vi "LS DAS Loop.vi"(11 "FPGA Ref":refnum<k20>) -> ()   [LabVIEW 2019]
uses:
  <vilib>/Utility/error.llb/Error Cluster From Error Code.vi
  <vilib>/rvi/errors/niLvFpgaAdjustHostInterfaceError.vi
  <vilib>/rvi/interface/nirviMethod/nirviMethod.xnode
  FPGA Bitfiles/LS_Acquisition_FPGA_9627.lvbitx
  <vilib>/rvi/errors/niLvFpgaMergeErrorWithErrorCode.vi
  <vilib>/FPGAPlugInAG/sbRIO-9627/niLvFpga_ReadFifo_sbRIO-9627.vi
panel:
  out "FIFO loops":i32
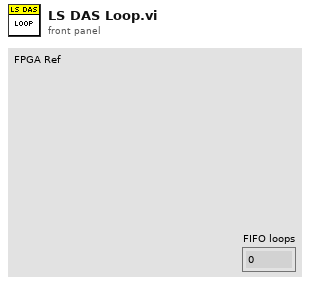
[diagram p1: front panel]
types:
  T1 = cluster{"FPGA Ref":refnum<k20>, "Time":dbl, "PtsTaken":i32, "Pts/File":i32, "10AveWait":u32, "Bank1 Filepath":path, "FileIndex":i32, "FilesUsed":i32, "Day":i32, "Bank2 Filepath":path, "DataCount":i32, "Note":string, "Anomaly Filepath":path, "File2 DataCount":i32}
  T2 = enum16{"Read", "Engine Writes", "Main Writes", "Write Anomalies", "Write Init Data", "Write Storage", "Write Note", "Read Note"}
  T3 = enum16{"open", "replace", "create", "open or create", "replace or create", "replace or create with confirmation"}
  T4 = typedef "LS Data.ctl" = cluster{"Total Cycles":u32[], "Steps":u32[], "Anomalies Total":i32[], "Cycles":u32[], "Anomalies/Cycle":i32[], "Anomalies (Last Cycle)":i32[], "Opens":i32[]}
  T5 = cluster{"Running?":bool, "Record":bool, "Data Filepath":path, "Serial Numbers":string[]}
  T6 = typedef "LVDateTimeRec.ctl" = cluster{"fractional second":dbl, "second":i32, "minute":i32, "hour":i32, "day of month":i32, "month":i32, "year":i32, "day of week":i32, "day of year":i32, "DST":i32}
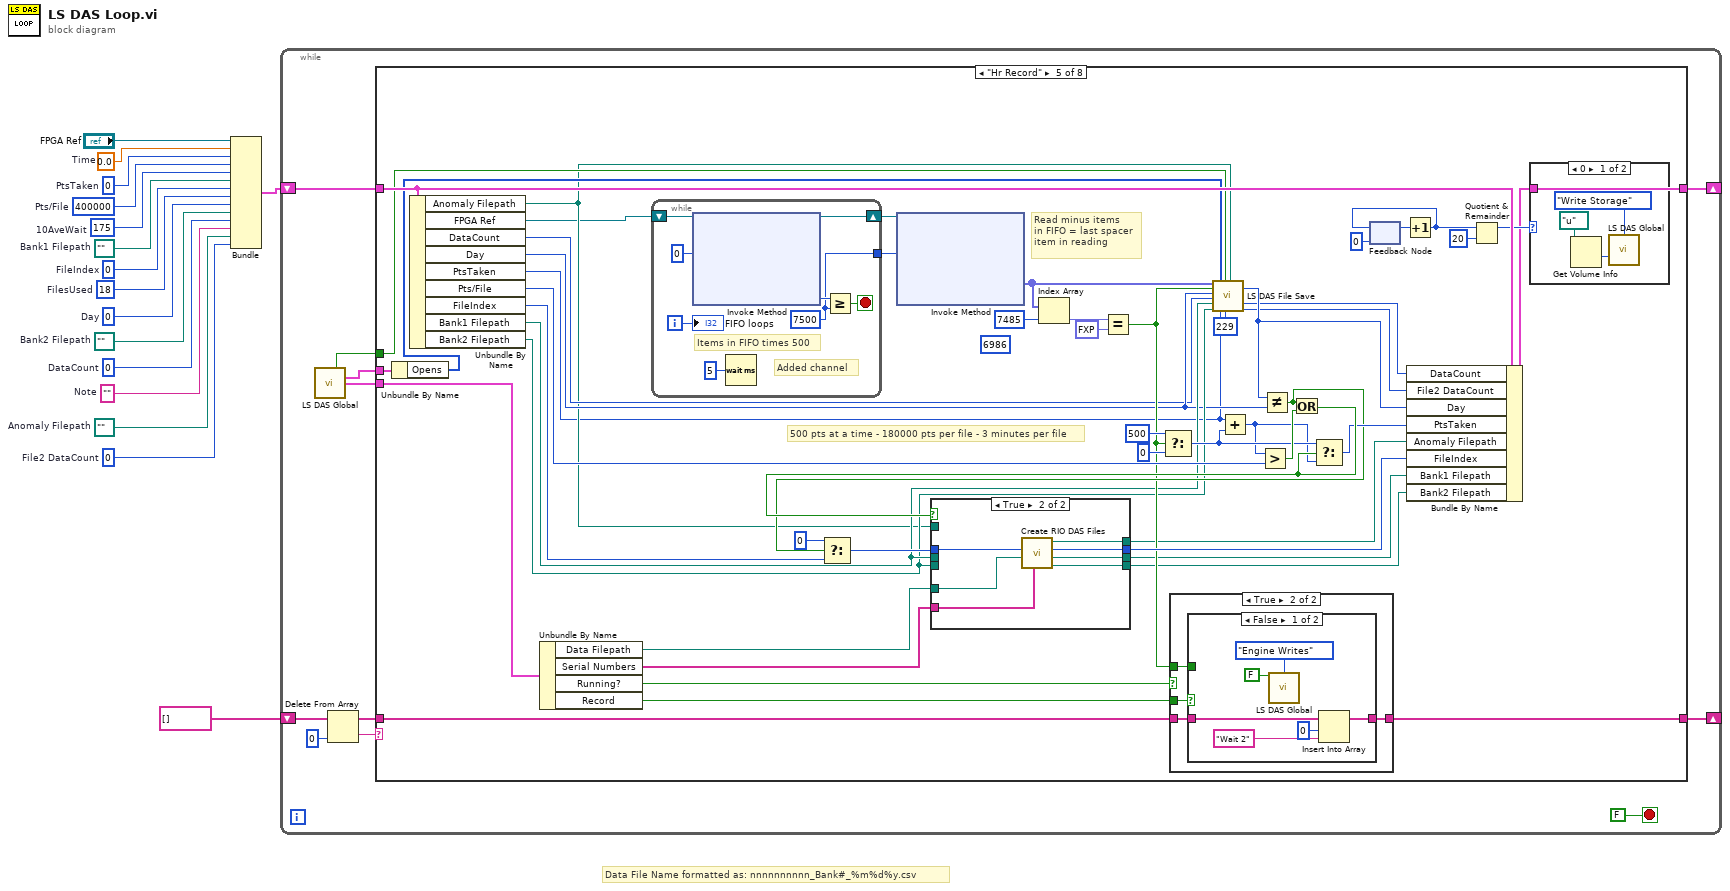
[diagram p0: block diagram]
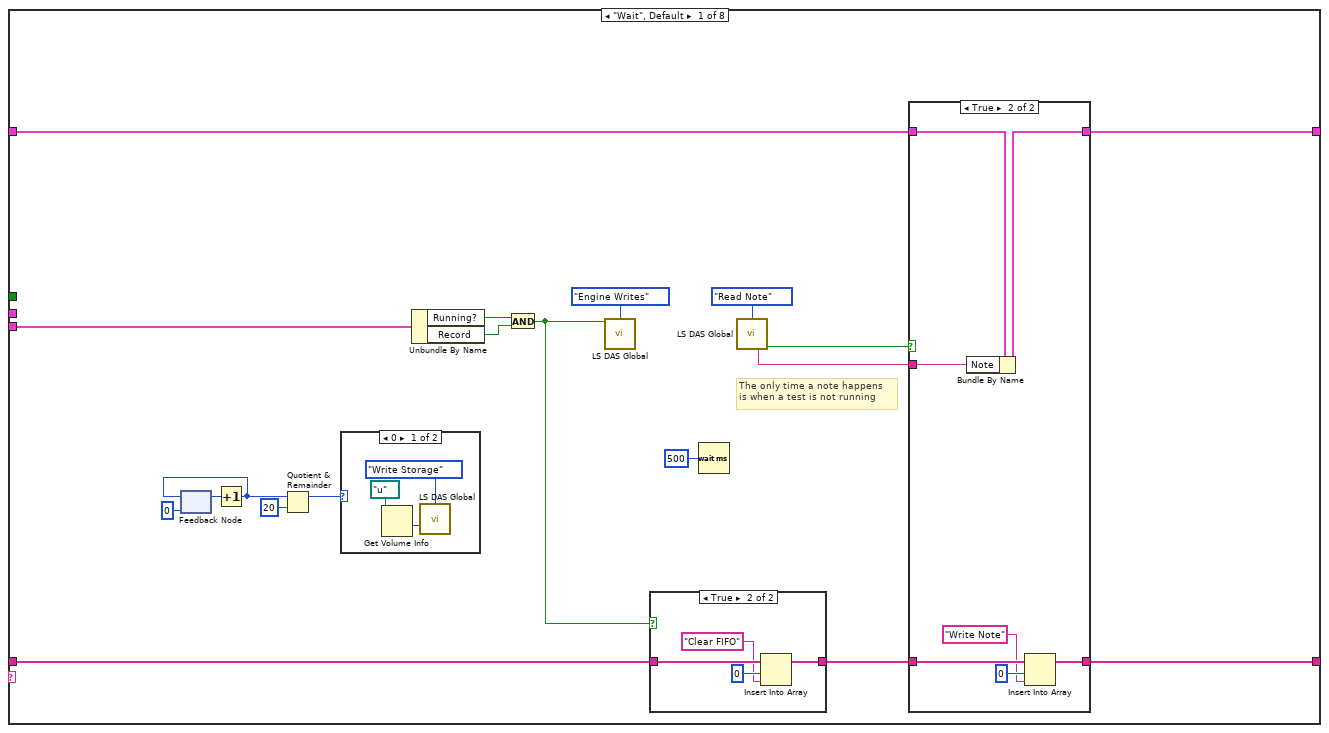
[diagram p2: hidden frame]
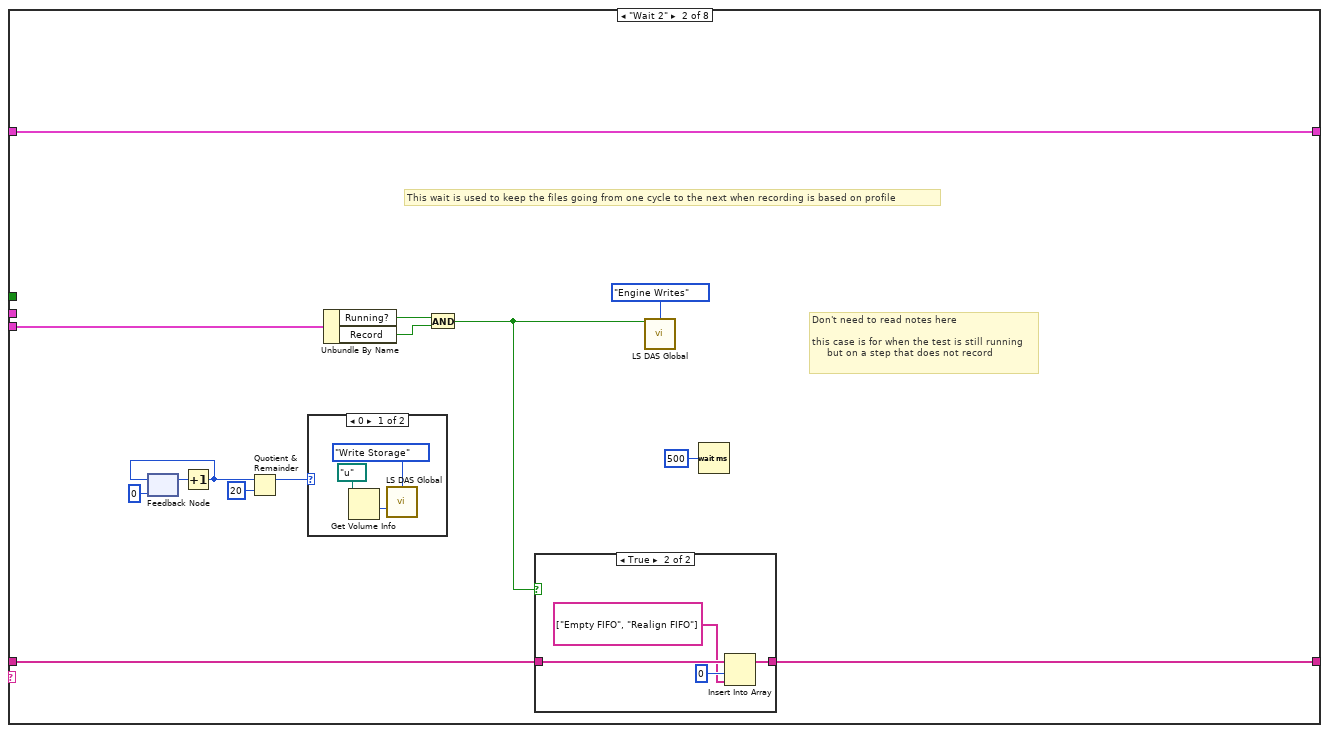
[diagram p6: hidden frame]
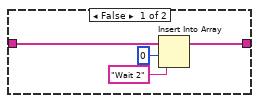
[diagram p8: hidden frame]
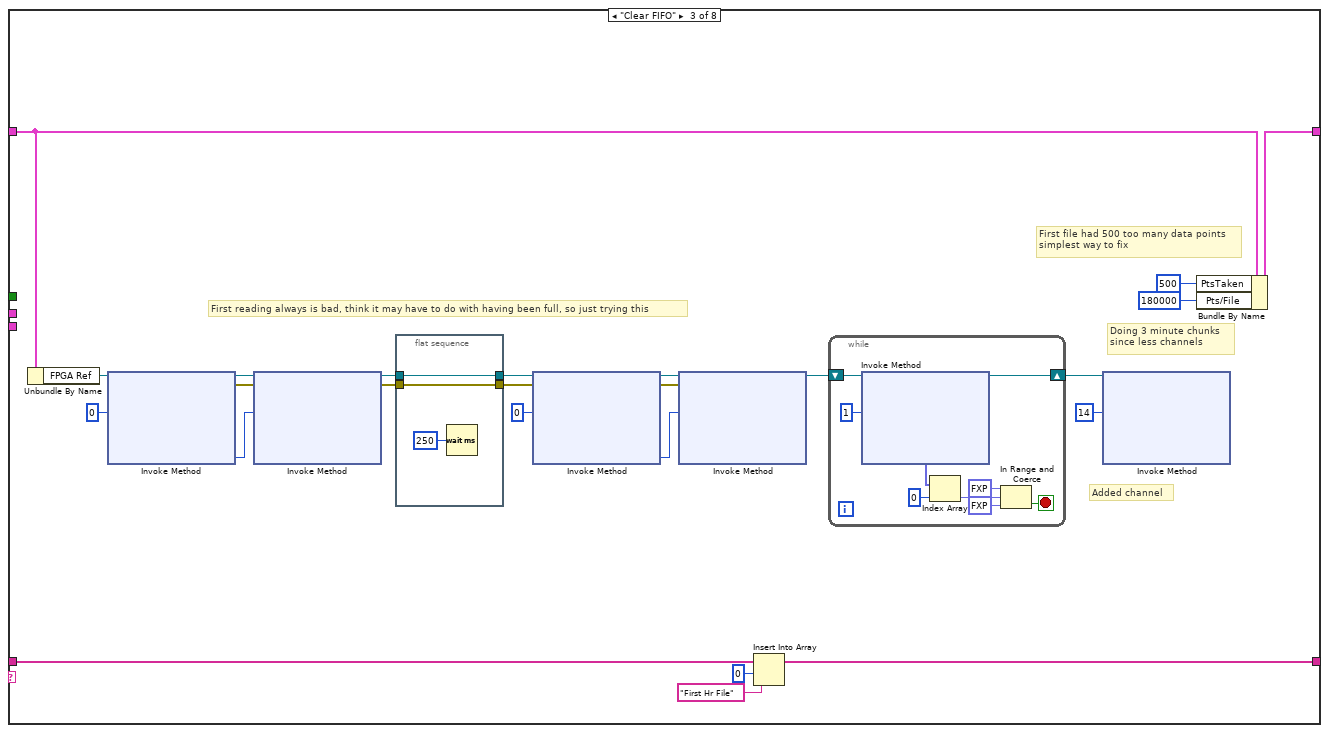
[diagram p9: hidden frame]
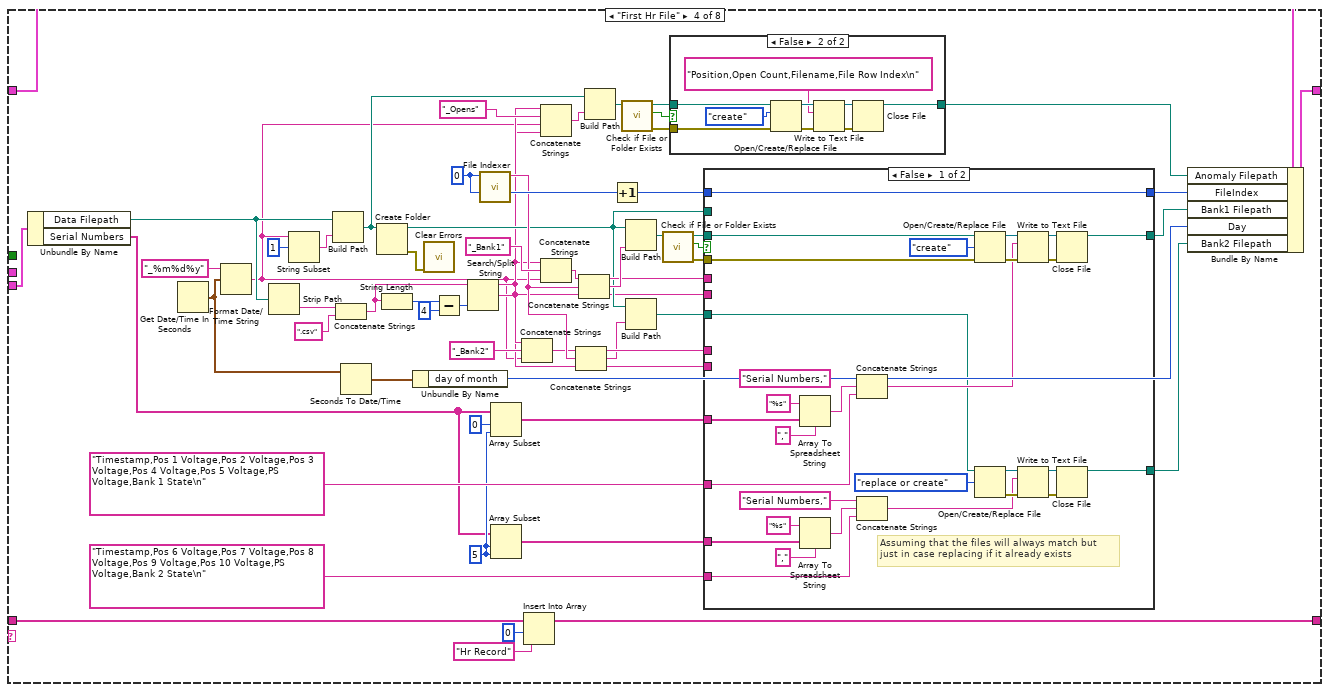
[diagram p10: hidden frame]
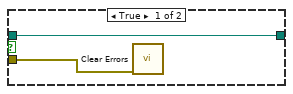
[diagram p11: hidden frame]
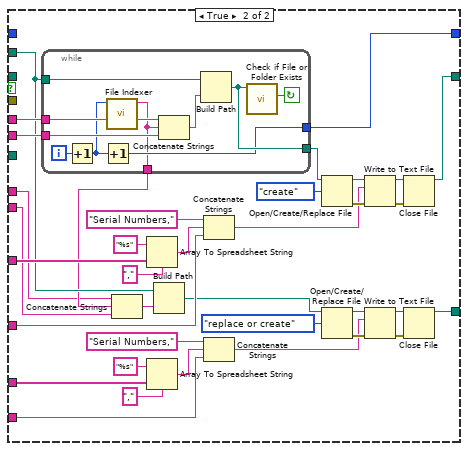
[diagram p12: hidden frame]
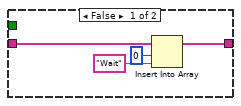
[diagram p14: hidden frame]
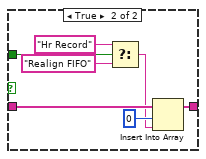
[diagram p15: hidden frame]
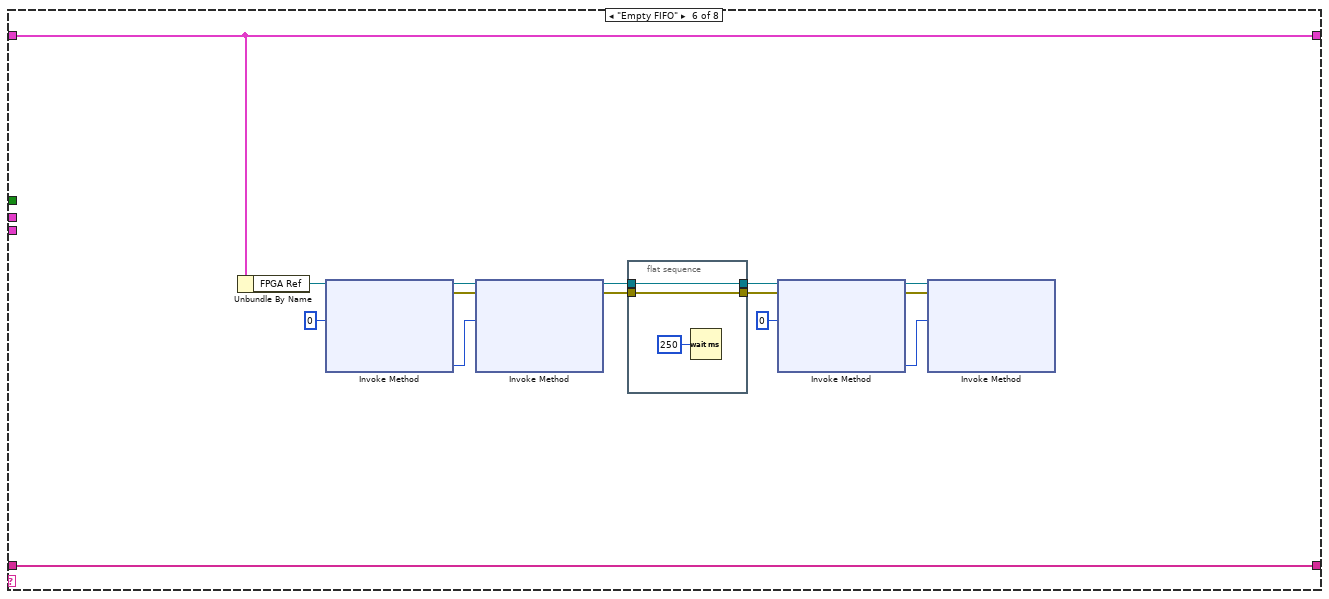
[diagram p17: hidden frame]
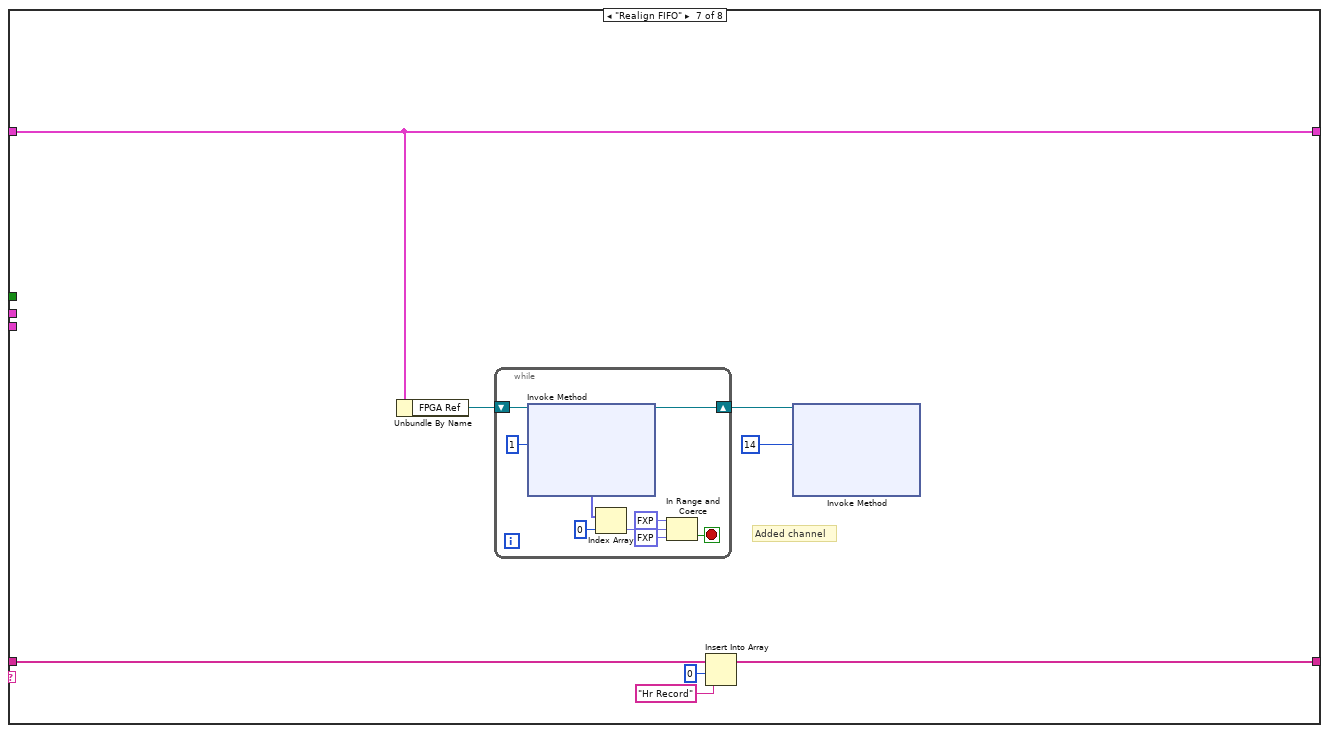
[diagram p18: hidden frame]
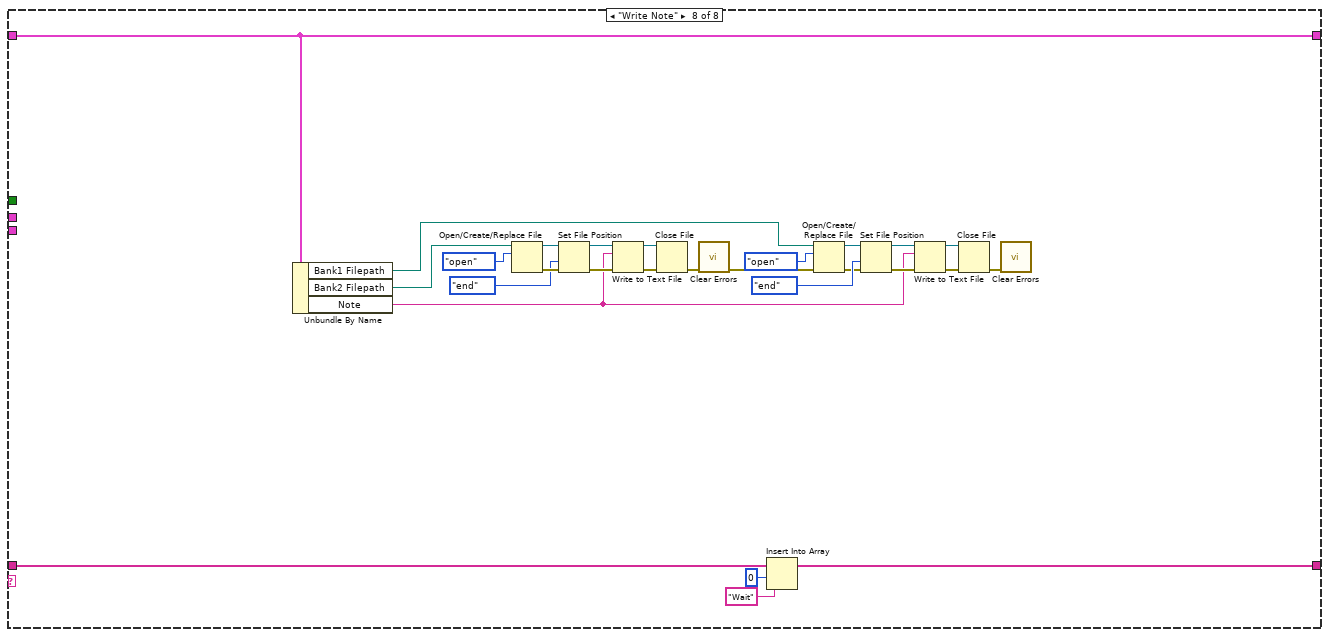
[diagram p19: hidden frame]
diagram:
  w2 = 0  # File2 DataCount
  w3 = path ""  # Anomaly Filepath
  w4 = ""  # Note
  w5 = 0  # DataCount
  w6 = path ""  # Bank2 Filepath
  w7 = 0  # Day
  w8 = 18  # FilesUsed
  w9 = 0  # FileIndex
  w10 = path ""  # Bank1 Filepath
  w11 = u32 175  # 10AveWait
  w12 = 400000  # Pts/File
  w13 = 0  # PtsTaken
  w16 = 0.0  # Time
  # "Data File Name formatted as: nnnnnnnnnn_Bank#_%m%d%y.csv"
  n1 = Bundle("FPGA Ref"="FPGA Ref", "Time"=w16, "PtsTaken"=w13, "Pts/File"=w12, "10AveWait"=w11, "Bank1 Filepath"=w10, "FileIndex"=w9, "FilesUsed"=w8, "Day"=w7, "Bank2 Filepath"=w6, "DataCount"=w5, "Note"=w4, "Anomaly Filepath"=w3, "File2 DataCount"=w2) -> (w15:T1)  [unwired: 1 in]
  n2 = while {
    shift-right: [w25] -> _
    shift-left: w15 -> [w26]
    shift-right: [w23] -> _
    shift-left: string[] [] -> [w24]
    stop <- FALSE stop-if-true
    n3 = call "LS DAS Global.vi"() -> ("Bank2Slow Out"=w17:bool, "Initial LS Data Out"=w19:T4, "LS Cluster Out"=w18:T5)  [unwired: 9 in, 4 out]
    n4 = Delete From Array(array=w24, index=0) -> (deleted portion=w21:string, array with subset deleted=w20:string[])  [unwired: 1 in]
    n5 = case shown="\"Hr Record\"" w21 {
      tunnel: w20 -> [w43 w74 w107 w179 w304 w376 w382 w424]
      tunnel: [w39 w73 w105 w178 w303 w376 w381 w423] -> w23
      tunnel: w18 -> [w44 w75 _ w181 w319 _ _ _]
      tunnel: w26 -> [w37 w72 w103 w130 w313 w377 w385 w420]
      tunnel: [w36 w72 w102 w180 w273 w377 w385 w420] -> w25
      tunnel: w19 -> [_ _ _ _ w283 _ _ _]
      tunnel: w17 -> [_ _ _ _ w282 _ _ _]
      frame "Wait", Default {
        # "The only time a note happens\nis when a test is not running"
        n6 = feedback #1(0) -> (w31:i32)
        n7 = Increment(x=w31) -> (x+1=w30:i32)
        n8 = feedback-in #1(w30) -> ()
        n9 = Quotient & Remainder(x=w30, y=20) -> (x-y*floor(x/y)=w28:i32)  [unwired: 1 out]
        n10 = case shown="0" w28 {
          frame 0 {
            n11 = Get Volume Info(11:path "u:/" ("path")) -> (1:w49:i64)  [unwired: 1 in, 5 out]
            n12 = call "LS DAS Global.vi"("Mode"=T2."Write Storage", "SDfree"=w49) -> ()  [unwired: 7 in, 7 out]
          }
          frame Default {
          }
        }
        n13 = Unbundle By Name(w44) -> ("Running?"=w45:bool, "Record"=w41:bool)
        n14 = And(x=w45, y=w41) -> (x .and. y?=w42:bool)
        n15 = call "LS DAS Global.vi"("Recording In"=w42, "Mode"=T2."Engine Writes") -> ()  [unwired: 7 in, 7 out]
        n16 = case shown="True" w42 {
          tunnel: w43 -> [w59 w63]
          tunnel: [w59 w62] -> w40
          frame False {
          }
          frame True {
            n17 = Insert Into Array(array=w63, index=0, new element="Clear FIFO" ("new element/subarray")) -> (w62:string[])
          }
        }
        n18 = Wait (ms)(milliseconds to wait=u32 500) -> ()  [unwired: 1 out]
        n19 = call "LS DAS Global.vi"("Mode"=T2."Read Note") -> ("Note Out"=w35:string, "Note Active"=w38:bool)  [unwired: 8 in, 5 out]
        n20 = case shown="True" w38 {
          tunnel: w40 -> [w51 w58]
          tunnel: [w51 w57] -> w39
          tunnel: w37 -> [w50 w54]
          tunnel: [w50 w53] -> w36
          tunnel: w35 -> [_ w55]
          frame False {
          }
          frame True {
            n21 = Bundle By Name(cluster=w54, "Note"=w55) -> (w53:T1)
            n22 = Insert Into Array(array=w58, index=0, new element="Write Note" ("new element/subarray")) -> (w57:string[])
          }
        }
      }
      frame "Wait 2" {
        # "Don't need to read notes here\n\nthis case is for when the test is still running\n     but on a step that does not record"
        # "This wait is used to keep the files going from one cycle to the next when recording is based on profile"
        n23 = feedback #2(0) -> (w67:i32)
        n24 = Increment(x=w67) -> (x+1=w66:i32)
        n25 = feedback-in #2(w66) -> ()
        n26 = Quotient & Remainder(x=w66, y=20) -> (x-y*floor(x/y)=w64:i32)  [unwired: 1 out]
        n27 = case shown="0" w64 {
          frame 0 {
            n28 = Get Volume Info(11:path "u:/" ("path")) -> (1:w80:i64)  [unwired: 1 in, 5 out]
            n29 = call "LS DAS Global.vi"("Mode"=T2."Write Storage", "SDfree"=w80) -> ()  [unwired: 7 in, 7 out]
          }
          frame Default {
          }
        }
        n30 = Unbundle By Name(w75) -> ("Running?"=w76:bool, "Record"=w70:bool)
        n31 = And(x=w76, y=w70) -> (x .and. y?=w71:bool)
        n32 = case shown="True" w71 {
          tunnel: w74 -> [w84 w88]
          tunnel: [w83 w87] -> w73
          frame False {
            n33 = Insert Into Array(array=w84, index=0, new element="Wait 2" ("new element/subarray")) -> (w83:string[])
          }
          frame True {
            n34 = Insert Into Array(array=w88, index=0, new element=string[] ["Empty FIFO", "Realign FIFO"]) -> (w87:string[])
          }
        }
        n35 = call "LS DAS Global.vi"("Recording In"=w71, "Mode"=T2."Engine Writes") -> ()  [unwired: 7 in, 7 out]
        n36 = Wait (ms)(milliseconds to wait=u32 500) -> ()  [unwired: 1 out]
      }
      frame "Clear FIFO" {
        # "First file had 500 too many data points\nsimplest way to fix"
        # "Doing 3 minute chunks\nsince less channels"
        # "First reading always is bad, think it may have to do with having been full, so just trying this"
        # "Added channel"
        n37 = Unbundle By Name(w103) -> ("FPGA Ref"=w112:refnum<k20>)
        n38 = xnode "Invoke Method"("FPGA VI Reference In"=w112, "Number of Elements"=u32 0) -> ("FPGA VI Reference Out"=w111:refnum<k20>, "error out"=w110:errorcluster, "Elements Remaining"=w108:u32)  [unwired: 2 in, 1 out]
        n39 = xnode "Invoke Method"("FPGA VI Reference In"=w111, "error in"=w110, "Number of Elements"=w108) -> ("FPGA VI Reference Out"=w92:refnum<k20>, "error out"=w91:errorcluster)  [unwired: 1 in, 2 out]
        n40 = flat-sequence {
          tunnel: w92 -> [w115]
          tunnel: w91 -> [w114]
          tunnel: [w115] -> w90
          tunnel: [w114] -> w89
          frame #0 {
            n41 = Wait (ms)(milliseconds to wait=u32 250) -> ()  [unwired: 1 out]
          }
        }
        n42 = xnode "Invoke Method"("FPGA VI Reference In"=w90, "error in"=w89, "Number of Elements"=u32 0) -> ("FPGA VI Reference Out"=w94:refnum<k20>, "error out"=w95:errorcluster, "Elements Remaining"=w97:u32)  [unwired: 1 in, 1 out]
        n43 = xnode "Invoke Method"("FPGA VI Reference In"=w94, "error in"=w95, "Number of Elements"=w97) -> ("FPGA VI Reference Out"=w93:refnum<k20>)  [unwired: 1 in, 3 out]
        n44 = Insert Into Array(array=w107, index=0, new element="First Hr File" ("new element/subarray")) -> (w105:string[])
        n45 = while {
          shift-right: [w123] -> w98
          shift-left: w93 -> [w124]
          stop <- w116 stop-if-true
          n46 = xnode "Invoke Method"("FPGA VI Reference In"=w124, "Number of Elements"=u32 1) -> ("FPGA VI Reference Out"=w123:refnum<k20>, "Data"=w121:fxp<+/-,22,11>[])  [unwired: 2 in, 2 out]
          n47 = Index Array(array=w121, index=0) -> (element=w119:fxp<+/-,22,11>)
          n48 = In Range and Coerce(upper limit=fxp<+/-,18,5> -14.0, x=w119, lower limit=fxp<+/-,18,5> -15.0) -> (In Range?=w116:bool)  [unwired: 1 out]
        }
        n49 = xnode "Invoke Method"("FPGA VI Reference In"=w98, "Number of Elements"=u32 14) -> ()  [unwired: 2 in, 4 out]
        n50 = Bundle By Name(cluster=w103, "PtsTaken"=500, "Pts/File"=180000 ("PtsNeeded")) -> (w102:T1)
      }
      frame "First Hr File" {
        w147 = 5 ("length")
        w153 = 0
        n51 = Unbundle By Name(w181) -> ("Data Filepath"=w162:path, "Serial Numbers"=w144:string[])
        n52 = Get Date/Time In Seconds() -> (seconds since 1Jan1904=w154:timestamp)
        n53 = Format Date/Time String(time format string (%c)="_%m%d%y", seconds (now)=w154) -> (date/time string=w125:string)  [unwired: 1 in]
        n54 = Strip Path(path=w162) -> (name=w173:string)  [unwired: 1 out]
        n55 = String Subset(string=w125, offset (0)=1) -> (substring=w171:string)  [unwired: 1 in]
        n56 = Build Path(base path=w162, name or relative path=w171) -> (appended path=w128:path)
        n57 = Concatenate Strings(w173, ".csv" ("string")) -> (w175:string)
        n58 = Seconds To Date/Time(time stamp (now)=w154) -> (date time rec=w155:T6)  [unwired: 1 in]
        n59 = Create Folder(path (use dialog)=w128) -> (created path=w138:path, error out=w161:errorcluster)  [unwired: 2 in, 1 out]
        n60 = String Length(string=w175) -> (length=w167:i32)
        n61 = Unbundle By Name(w155) -> ("day of month"=w152:i32)
        n62 = call <vilib>:"Clear Errors.vi"("error in (no error)"=w161) -> ()  [unwired: 5 in, 2 out]
        n63 = Subtract(x=w167, y=4) -> (x-y=w169:i32)
        n64 = Search/Split String(string=w175, offset (0)=w169) -> (substring before match=w127:string, match + rest of string=w126:string)  [unwired: 1 in, 1 out]
        n65 = call "File Indexer.vi"("File Index In"=w153) -> ("File Indicator Out"=w141:string)  [unwired: 10 in]
        n66 = Array Subset(array=w144, index=0, length=w147) -> (w148:string[])
        n67 = Array Subset(array=w144, index=w147, length=w147) -> (w145:string[])
        n68 = Concatenate Strings(w127, "_Bank2" ("string"), w125) -> (w140:string)
        n69 = Insert Into Array(array=w179, index=0, new element="Hr Record" ("new element/subarray")) -> (w178:string[])
        n70 = Concatenate Strings(w127, "_Opens" ("string"), w125, w126) -> (w132:string)
        n71 = Concatenate Strings(w127, "_Bank1" ("string"), w125) -> (w156:string)
        n72 = Concatenate Strings(w140, w141, w126) -> (w139:string)
        n73 = Concatenate Strings(w156, w141, w126) -> (w157:string)
        n74 = Build Path(base path=w128, name or relative path=w132) -> (appended path=w131:path)
        n75 = Increment(x=w153) -> (x+1=w159:i32)
        n76 = call <vilib>:"Check if File or Folder Exists.vi"("path"=w131) -> ("error out"=w135:errorcluster, "file or folder exists?"=w136:bool, "dup path"=w134:path)  [unwired: 8 in]
        n77 = Build Path(base path=w138, name or relative path=w157) -> (appended path=w166:path)
        n78 = Build Path(base path=w138, name or relative path=w139) -> (appended path=w137:path)
        n79 = call <vilib>:"Check if File or Folder Exists.vi"("path"=w166) -> ("error out"=w163:errorcluster, "file or folder exists?"=w165:bool, "dup path"=w164:path)  [unwired: 8 in]
        n80 = case shown="False" w136 {
          tunnel: w134 -> [w183 w188]
          tunnel: w135 -> [w182 w187]
          tunnel: [w183 w184] -> w129
          frame True {
            n81 = call <vilib>:"Clear Errors.vi"("error in (no error)"=w182) -> ()  [unwired: 5 in, 2 out]
          }
          frame False {
            n82 = Open/Create/Replace File(file path (use dialog)=w188, error in=w187, operation (0:open)=T3."create") -> (refnum out=w191:refnum<file>, error out=w189:errorcluster)  [unwired: 3 in, 1 out]
            n83 = Write to Text File(file (use dialog)=w191, text="Position,Open Count,Filename,File Row Index\n", error in=w189) -> (refnum out=w192:refnum<file>, error out=w190:errorcluster)  [unwired: 1 in, 1 out]
            n84 = Close File(refnum=w192, error in=w190) -> (path=w184:path)  [unwired: 1 out]
          }
        }
        n85 = case shown="False" w165 {
          tunnel: w164 -> [w217 _]
          tunnel: [w216 w244] -> w160
          tunnel: w163 -> [w215 _]
          tunnel: w148 -> [w210 w251]
          tunnel: w159 -> [w208 _]
          tunnel: [w208 w256] -> w158
          tunnel: w156 -> [_ w258]
          tunnel: w126 -> [_ w257]
          tunnel: w138 -> [_ w227]
          tunnel: "Timestamp,Pos 1 Voltage,Pos 2 Voltage,Pos 3 Voltage,Pos 4 Voltage,Pos 5 Voltage,PS Voltage,Bank 1 State\n" -> [w207 w242]
          tunnel: "Timestamp,Pos 6 Voltage,Pos 7 Voltage,Pos 8 Voltage,Pos 9 Voltage,Pos 10 Voltage,PS Voltage,Bank 2 State\n" -> [w201 w237]
          tunnel: [w195 w230] -> w149
          tunnel: w145 -> [w202 w229]
          tunnel: w140 -> [_ w224]
          tunnel: w126 -> [_ w223]
          tunnel: w137 -> [w193 _]
          frame False {
            # "Assuming that the files will always match but\njust in case replacing if it already exists"
            n86 = Array To Spreadsheet String(delimiter (Tab)=",", array=w210, 3:"%s" ("format string")) -> (spreadsheet string=w211:string)
            n87 = Array To Spreadsheet String(delimiter (Tab)=",", array=w202, 3:"%s" ("format string")) -> (spreadsheet string=w206:string)
            n88 = Concatenate Strings("Serial Numbers," ("string"), w211, w207) -> (w209:string)
            n89 = Concatenate Strings("Serial Numbers," ("string"), w206, w201) -> (w194:string)
            n90 = Open/Create/Replace File(file path (use dialog)=w217, error in=w215, operation (0:open)=T3."create") -> (refnum out=w219:refnum<file>, error out=w221:errorcluster)  [unwired: 3 in, 1 out]
            n91 = Open/Create/Replace File(file path (use dialog)=w193, operation (0:open)=T3."replace or create") -> (refnum out=w199:refnum<file>, error out=w197:errorcluster)  [unwired: 4 in, 1 out]
            n92 = Write to Text File(file (use dialog)=w219, text=w209, error in=w221) -> (refnum out=w218:refnum<file>, error out=w220:errorcluster)  [unwired: 1 in, 1 out]
            n93 = Write to Text File(file (use dialog)=w199, text=w194, error in=w197) -> (refnum out=w200:refnum<file>, error out=w198:errorcluster)  [unwired: 1 in, 1 out]
            n94 = Close File(refnum=w218, error in=w220) -> (path=w216:path)  [unwired: 1 out]
            n95 = Close File(refnum=w200, error in=w198) -> (path=w195:path)  [unwired: 1 out]
          }
          frame True {
            n96 = while {
              tunnel: w227 -> [w268]
              tunnel: w258 -> [w267]
              tunnel: w257 -> [w266]
              tunnel: [w263] -> w245
              tunnel: [w261] -> w256
              tunnel: [w259] -> w225
              i -> [w262]
              stop <- w264 continue-if-true
              n97 = Increment(x=w262) -> (x+1=w260:i32)
              n98 = Increment(x=w260) -> (x+1=w261:i32)
              n99 = call "File Indexer.vi"("File Index In"=w260) -> ("File Indicator Out"=w259:string)  [unwired: 10 in]
              n100 = Concatenate Strings(w267, w259, w266) -> (w265:string)
              n101 = Build Path(base path=w268, name or relative path=w265) -> (appended path=w263:path)
              n102 = call <vilib>:"Check if File or Folder Exists.vi"("path"=w263) -> ("file or folder exists?"=w264:bool)  [unwired: 8 in, 2 out]
            }
            n103 = Concatenate Strings(w224, w225, w223) -> (w226:string)
            n104 = Array To Spreadsheet String(delimiter (Tab)=",", array=w251, 3:"%s" ("format string")) -> (spreadsheet string=w252:string)
            n105 = Array To Spreadsheet String(delimiter (Tab)=",", array=w229, 3:"%s" ("format string")) -> (spreadsheet string=w241:string)
            n106 = Build Path(base path=w227, name or relative path=w226) -> (appended path=w228:path)
            n107 = Concatenate Strings("Serial Numbers," ("string"), w252, w242) -> (w243:string)
            n108 = Concatenate Strings("Serial Numbers," ("string"), w241, w237) -> (w233:string)
            n109 = Open/Create/Replace File(file path (use dialog)=w245, operation (0:open)=T3."create") -> (refnum out=w247:refnum<file>, error out=w249:errorcluster)  [unwired: 4 in, 1 out]
            n110 = Open/Create/Replace File(file path (use dialog)=w228, operation (0:open)=T3."replace or create") -> (refnum out=w232:refnum<file>, error out=w235:errorcluster)  [unwired: 4 in, 1 out]
            n111 = Write to Text File(file (use dialog)=w247, text=w243, error in=w249) -> (refnum out=w246:refnum<file>, error out=w248:errorcluster)  [unwired: 1 in, 1 out]
            n112 = Write to Text File(file (use dialog)=w232, text=w233, error in=w235) -> (refnum out=w231:refnum<file>, error out=w236:errorcluster)  [unwired: 1 in, 1 out]
            n113 = Close File(refnum=w246, error in=w248) -> (path=w244:path)  [unwired: 1 out]
            n114 = Close File(refnum=w231, error in=w236) -> (path=w230:path)  [unwired: 1 out]
          }
        }
        n115 = Bundle By Name(cluster=w130, "Anomaly Filepath"=w129, "FileIndex"=w158, "Bank1 Filepath"=w160, "Day"=w152, "Bank2 Filepath"=w149) -> (w180:T1)
      }
      frame "Hr Record" {
        (unwired) 6986 ("index")
        # "Read minus items\nin FIFO = last spacer\nitem in reading"
        # "500 pts at a time - 180000 pts per file - 3 minutes per file"
        n116 = Unbundle By Name(w283) -> ("Opens"=w281:i32[])
        n117 = Unbundle By Name(w313) -> ("Anomaly Filepath"=w279:path, "FPGA Ref"=w272:refnum<k20>, "DataCount"=w284:i32, "Day"=w285:i32, "PtsTaken"=w269:i32, "Pts/File"=w312:i32, "FileIndex"=w296:i32, "Bank1 Filepath"=w288:path, "Bank2 Filepath"=w287:path)
        n118 = Unbundle By Name(w319) -> ("Data Filepath"=w302:path, "Serial Numbers"=w307:string[], "Running?"=w306:bool, "Record"=w305:bool)
        n119 = while {
          tunnel: [w360] -> w318
          shift-right: [w357] -> w317
          shift-left: w272 -> [w358]
          i -> [w356]
          stop <- w359 stop-if-true
          w360 = u32 7500 ("y")
          # "Added channel"
          # "Items in FIFO times 500"
          n120 = xnode "Invoke Method"("FPGA VI Reference In"=w358, "Number of Elements"=u32 0) -> ("FPGA VI Reference Out"=w357:refnum<k20>, "Elements Remaining"=w361:u32)  [unwired: 2 in, 2 out]
          n121 = Wait (ms)(milliseconds to wait=u32 5) -> ()  [unwired: 1 out]
          n122 = Greater Or Equal?(x=w361, y=w360) -> (x >= y?=w359:bool)
          "FIFO loops" <- w356
        }
        n123 = xnode "Invoke Method"("FPGA VI Reference In"=w317, "Number of Elements"=w318) -> ("Data"=w293:fxp<+/-,22,11>[])  [unwired: 2 in, 3 out]
        n124 = Index Array(array=w293, index=7485) -> (element=w311:fxp<+/-,22,11>)
        n125 = Equal?(x=w311, y=fxp<+/-,18,5> -15.0) -> (x = y?=w292:bool)
        n126 = Select(t=500 ("PtsTaken"), s=w292, f=0 ("PtsTaken")) -> (s? t:f=w300:i32)
        n127 = case shown="True" w306 {
          tunnel: w304 -> [w325 w330]
          tunnel: [w324 w329] -> w303
          tunnel: w292 -> [_ w327]
          tunnel: w305 -> [_ w328]
          frame False {
            n128 = Insert Into Array(array=w325, index=0, new element="Wait") -> (w324:string[])
          }
          frame True {
            n129 = case shown="False" w328 {
              tunnel: w330 -> [w336 w343]
              tunnel: [w335 w342] -> w329
              tunnel: w327 -> [_ w340]
              frame False {
                n130 = call "LS DAS Global.vi"("Recording In"=FALSE, "Mode"=T2."Engine Writes") -> ()  [unwired: 7 in, 7 out]
                n131 = Insert Into Array(array=w336, index=0, new element="Wait 2") -> (w335:string[])
              }
              frame True {
                n132 = Select(t="Hr Record", s=w340, f="Realign FIFO" ("new element/subarray")) -> (s? t:f=w338:string)
                n133 = Insert Into Array(array=w343, index=0, new element=w338) -> (w342:string[])
              }
            }
          }
        }
        n134 = call "LS DAS File Save.vi"("Raw Data"=w293, "ValidFifoRead"=w292, "Day In"=w285, "Count In"=w284, "Bank1 Filepath"=w288, "Bank2 Filepath"=w287, "Opens In"=w281, "Row Count In"=w269, "Bank2Slow"=w282, "LowRate"=229, "Anomaly Filepath"=w279) -> ("Day Out"=w291:i32, "Count Out"=w271:i32, "Second File Count Out"=w270:i32)  [unwired: 6 in]
        n135 = Add(x=w269, y=w300) -> (x+y=w299:i32)
        n136 = Greater?(x=w299, y=w312) -> (0:w309:bool)
        n137 = Not Equal?(x=w291, y=w285) -> (x != y?=w297:bool)
        n138 = Select(t=0, s=w297, f=w296) -> (s? t:f=w295:i32)
        n139 = Or(x=w297, y=w309) -> (x .or. y?=w301:bool)
        n140 = case shown="True" w301 {
          tunnel: w288 -> [w347 _]
          tunnel: [w347 w350] -> w290
          tunnel: w295 -> [w346 w354]
          tunnel: [w346 w351] -> w308
          tunnel: w307 -> [_ w352]
          tunnel: w302 -> [_ w353]
          tunnel: [w345 w349] -> w289
          tunnel: w287 -> [w345 _]
          tunnel: [w344 w348] -> w280
          tunnel: w279 -> [w344 _]
          frame False {
          }
          frame True {
            n141 = call "Create RIO DAS Files.vi"("Serial Numbers"=w352, "Base Filepath"=w353, "File Index In"=w354) -> ("Bank2 Filepath"=w349:path, "Bank1 Filepath"=w350:path, "File Index Out"=w351:i32, "Anomaly Filepath"=w348:path)  [unwired: 5 in]
          }
        }
        n142 = Select(t=w300, s=w301, f=w299) -> (s? t:f=w298:i32)
        n143 = feedback #3(0) -> (w277:i32)
        n144 = Increment(x=w277) -> (x+1=w276:i32)
        n145 = feedback-in #3(w276) -> ()
        n146 = Bundle By Name(cluster=w313, "DataCount"=w271, "File2 DataCount"=w270, "Day"=w291, "PtsTaken"=w298, "Anomaly Filepath"=w280, "FileIndex"=w308, "Bank1 Filepath"=w290, "Bank2 Filepath"=w289) -> (w273:T1)
        n147 = Quotient & Remainder(x=w276, y=20) -> (x-y*floor(x/y)=w274:i32)  [unwired: 1 out]
        n148 = case shown="0" w274 {
          tunnel: w273 -> [_ _]
          frame 0 {
            n149 = Get Volume Info(11:path "u:/" ("path")) -> (1:w322:i64)  [unwired: 1 in, 5 out]
            n150 = call "LS DAS Global.vi"("Mode"=T2."Write Storage", "SDfree"=w322) -> ()  [unwired: 7 in, 7 out]
          }
          frame Default {
          }
        }
      }
      frame "Empty FIFO" {
        n151 = Unbundle By Name(w377) -> ("FPGA Ref"=w375:refnum<k20>)
        n152 = xnode "Invoke Method"("FPGA VI Reference In"=w375, "Number of Elements"=u32 0) -> ("FPGA VI Reference Out"=w374:refnum<k20>, "error out"=w373:errorcluster, "Elements Remaining"=w371:u32)  [unwired: 2 in, 1 out]
        n153 = xnode "Invoke Method"("FPGA VI Reference In"=w374, "error in"=w373, "Number of Elements"=w371) -> ("FPGA VI Reference Out"=w366:refnum<k20>, "error out"=w365:errorcluster)  [unwired: 1 in, 2 out]
        n154 = flat-sequence {
          tunnel: w366 -> [w380]
          tunnel: w365 -> [w379]
          tunnel: [w380] -> w364
          tunnel: [w379] -> w363
          frame #0 {
            n155 = Wait (ms)(milliseconds to wait=u32 250) -> ()  [unwired: 1 out]
          }
        }
        n156 = xnode "Invoke Method"("FPGA VI Reference In"=w364, "error in"=w363, "Number of Elements"=u32 0) -> ("FPGA VI Reference Out"=w367:refnum<k20>, "error out"=w368:errorcluster, "Elements Remaining"=w370:u32)  [unwired: 1 in, 1 out]
        n157 = xnode "Invoke Method"("FPGA VI Reference In"=w367, "error in"=w368, "Number of Elements"=w370) -> ()  [unwired: 1 in, 4 out]
      }
      frame "Realign FIFO" {
        # "Added channel"
        n158 = Unbundle By Name(w385) -> ("FPGA Ref"=w388:refnum<k20>)
        n159 = while {
          shift-right: [w396] -> w386
          shift-left: w388 -> [w397]
          stop <- w389 stop-if-true
          n160 = xnode "Invoke Method"("FPGA VI Reference In"=w397, "Number of Elements"=u32 1) -> ("FPGA VI Reference Out"=w396:refnum<k20>, "Data"=w394:fxp<+/-,22,11>[])  [unwired: 2 in, 2 out]
          n161 = Index Array(array=w394, index=0) -> (element=w392:fxp<+/-,22,11>)
          n162 = In Range and Coerce(upper limit=fxp<+/-,18,5> -14.0, x=w392, lower limit=fxp<+/-,18,5> -15.0) -> (In Range?=w389:bool)  [unwired: 1 out]
        }
        n163 = Insert Into Array(array=w382, index=0, new element="Hr Record" ("new element/subarray")) -> (w381:string[])
        n164 = xnode "Invoke Method"("FPGA VI Reference In"=w386, "Number of Elements"=u32 14) -> ()  [unwired: 2 in, 4 out]
      }
      frame "Write Note" {
        n165 = Unbundle By Name(w420) -> ("Bank1 Filepath"=w400:path, "Bank2 Filepath"=w399:path, "Note"=w398:string)
        n166 = Open/Create/Replace File(file path (use dialog)=w399, operation (0:open)=T3."open") -> (refnum out=w415:refnum<file>, error out=w414:errorcluster)  [unwired: 4 in, 1 out]
        n167 = Set File Position(refnum=w415, from (0:start)=enum16{"start", "end", "current"}."end", error in=w414) -> (refnum out=w411:refnum<file>, error out=w412:errorcluster)  [unwired: 1 in]
        n168 = Write to Text File(file (use dialog)=w411, text=w398, error in=w412) -> (refnum out=w418:refnum<file>, error out=w419:errorcluster)  [unwired: 1 in, 1 out]
        n169 = Close File(refnum=w418, error in=w419) -> (error out=w417:errorcluster)  [unwired: 1 out]
        n170 = call <vilib>:"Clear Errors.vi"("error in (no error)"=w417) -> ("error out"=w401:errorcluster)  [unwired: 5 in, 1 out]
        n171 = Insert Into Array(array=w424, index=0, new element="Wait" ("new element/subarray")) -> (w423:string[])
        n172 = Open/Create/Replace File(file path (use dialog)=w400, error in=w401, operation (0:open)=T3."open") -> (refnum out=w406:refnum<file>, error out=w407:errorcluster)  [unwired: 3 in, 1 out]
        n173 = Set File Position(refnum=w406, from (0:start)=enum16{"start", "end", "current"}."end", error in=w407) -> (refnum out=w410:refnum<file>, error out=w409:errorcluster)  [unwired: 1 in]
        n174 = Write to Text File(file (use dialog)=w410, text=w398, error in=w409) -> (refnum out=w403:refnum<file>, error out=w402:errorcluster)  [unwired: 1 in, 1 out]
        n175 = Close File(refnum=w403, error in=w402) -> (error out=w404:errorcluster)  [unwired: 1 out]
        n176 = call <vilib>:"Clear Errors.vi"("error in (no error)"=w404) -> ()  [unwired: 5 in, 2 out]
      }
    }
  }
